vi "Loader Management Core.vi"(9 "Loader Name Override":string, 10 "Plugin Loader Path Override":path, 11 "CIFPluginManager in":refnum<class "CIFPluginManager.lvclass">) -> (0 "error out":errorcluster)   [LabVIEW 2021, in "CIFPluginManager.lvclass"]
uses:
  CIFPluginManager.lvclass
  CIFPluginManager.lvclass/CIFPluginManager.ctl
  typedef/Loader Load Command.ctl
  typedef/Loader Type.ctl
  CIFUtilities/CIFLogs/Logs/Write Error.vi
  gRPC/CIF_Manager_Client_Wrapper/CIFManagerClientWrapper.lvlib
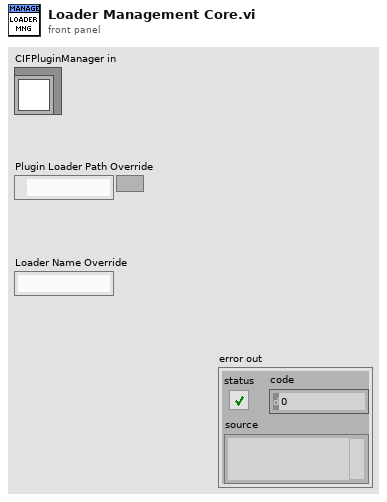
[diagram p1: front panel]
types:
  T1 = typedef "CIFPluginManager.lvclass/Loader Load Command.ctl" = cluster{"Loader Type":T2, "Loader Name":string}
  T2 = typedef "CIFPluginManager.lvclass/Loader Type.ctl" = enum16{"LabVIEW"}
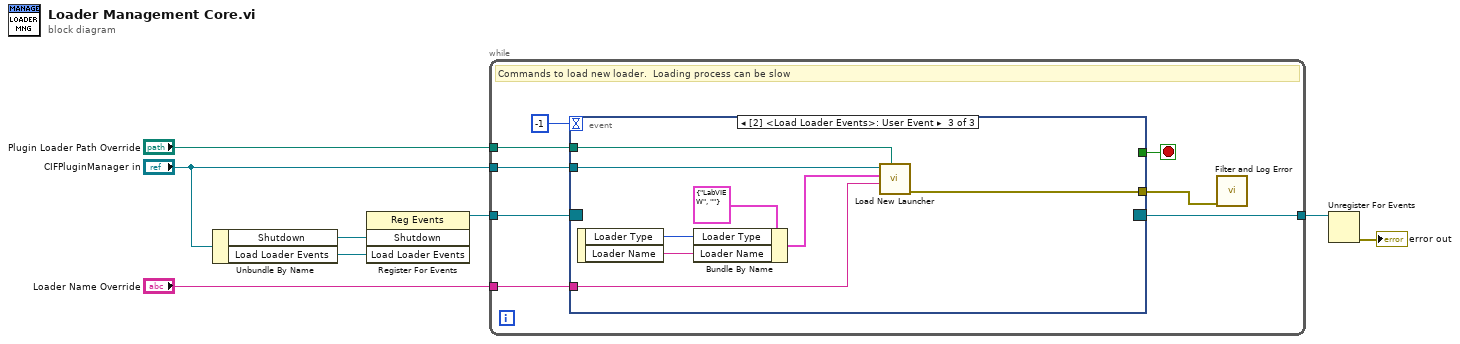
[diagram p0: block diagram]
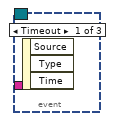
[diagram p2: hidden frame]
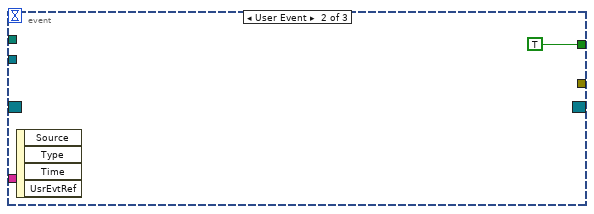
[diagram p3: hidden frame]
diagram:
  n1 = Unbundle By Name("CIFPluginManager in") -> ("Shutdown"=w5:refnum<user-event>, "Load Loader Events"=w6:refnum<user-event>)
  n2 = register-events(w5, w6) -> (reference out=w4:refnum<event-registration>)  [unwired: 2 in, 1 out]
  n3 = while {
    tunnel: w4 -> [w16]
    tunnel: [w12] -> w7
    tunnel: "Plugin Loader Path Override" -> [w10]
    tunnel: "Loader Name Override" -> [w9]
    tunnel: "CIFPluginManager in" -> [w15]
    stop <- w13 stop-if-true
    # "Commands to load new loader.  Loading process can be slow"
    n4 = event shown="[2] <Load Loader Events>: User Event" {
      selector: w16 -> [_ _ _]
      dyn-events: [_ _ _] -> w12
      timeout: -1 -> [_ _ _]
      tunnel: w15 -> [_ _ w25]
      tunnel: [_ TRUE _] -> w13
      tunnel: [_ _ w24] -> w11
      tunnel: w10 -> [_ _ w19]
      tunnel: w9 -> [_ _ w18]
      event Timeout {
        n5 = event-data() -> ()  [unwired: 1 in, 3 out]
      }
      event User Event {
        n6 = event-data() -> ()  [unwired: 1 in, 4 out]
      }
      event User Event {
        n7 = event-data() -> ("Loader Type"=w22:T2, "Loader Name"=w21:string)  [unwired: 1 in]
        n8 = Bundle By Name(cluster=T1 {"Loader Type"=enum."LabVIEW", "Loader Name"=""} ("Launcher Load Info"), "Loader Type"=w22, "Loader Name"=w21) -> (w20:T1)
        n9 = call "Load New Launcher.vi"("Plugin Loader Path Override"=w19, "Loader Name Override"=w18, "Loader Load Info"=w20, "CIFPluginManager in"=w25) -> ("error out"=w24:errorcluster)  [unwired: 7 in]
      }
    }
    n10 = call "Filter and Log Error.vi"("error In"=w11) -> ()  [unwired: 11 in]
  }
  n11 = Unregister For Events(event registration refnum=w7) -> (error out=→"error out":errorcluster)  [unwired: 1 in]
